vi "To-string-array.vi"(8 "error in (no error)":errorcluster, 11 "Action in":refnum<class "Move-Timer.lvclass">) -> (0 "error out":errorcluster, 2 "Action string array":string[](array[string]), 3 "Action out":refnum<class "Move-Timer.lvclass">)   [LabVIEW 2013, in "PowderDeposition.lvlib" / "Move-Timer.lvclass"]
uses:
  Move-Timer.lvclass
  Move-Timer.lvclass/Move-Timer.ctl
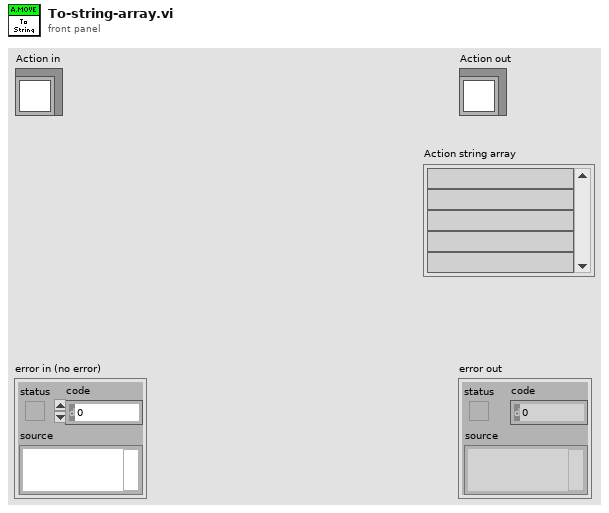
[diagram p1: front panel]
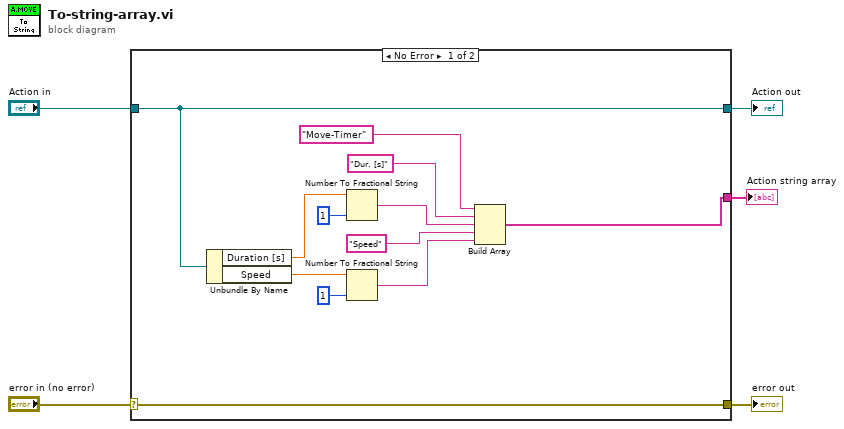
[diagram p0: block diagram]
diagram:
  n1 = case shown="No Error" "error in (no error)" {
    selector: "error in (no error)" -> [w17 w19]
    tunnel: [w17 w19] -> w4
    tunnel: [w16 w18] -> w2
    tunnel: "Action in" -> [w16 w18]
    tunnel: [w6 _] -> w1
    frame No Error {
      n2 = Unbundle By Name(w16) -> ("Duration [s]"=w15:dbl, "Speed"=w14:dbl)
      n3 = Number To Fractional String(number=w15, precision (6)=i16 1) -> (F-format string=w10:string)  [unwired: 2 in]
      n4 = Number To Fractional String(number=w14, precision (6)=i16 1) -> (F-format string=w8:string)  [unwired: 2 in]
      n5 = Build Array("Move-Timer", "Dur. [s]", w10, "Speed", w8) -> (w6:string[])
    }
    frame Error {
    }
  }
  "error out" <- w4
  "Action out" <- w2
  "Action string array" <- w1
